vi "MBDRV_Communication With Server.vi"(8 "error in (no error)":errorcluster, 11 "Write To PLC":T4) -> (0 "error out":errorcluster, 3 "Read From PLC":T1)   [LabVIEW 2010]
uses:
  SubVIs/ModBUS Driver/Private/MBDRV_Command List.ctl
  SubVIs/ModBUS Driver/Private/MBDRV_Command Data.ctl
  SubVIs/ModBUS Driver/Private/MBDRV_Action.ctl
  SubVIs/ModBUS Driver/Private/MBDRV_Response List.ctl
  SubVIs/ModBUS Driver/Private/MBDRV_Response.ctl
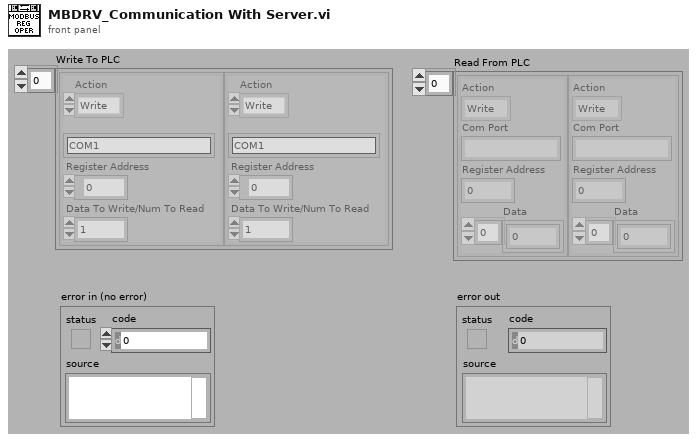
[diagram p1: front panel]
types:
  T1 = typedef "MBDRV_Response List.ctl" = T2[]
  T2 = typedef "MBDRV_Response.ctl" = cluster{"Action":T3, "Com Port":string, "Register Address":u16, "Data":i16[]}
  T3 = typedef "MBDRV_Action.ctl" = enum16{"Write", "Read"}
  T4 = typedef "MBDRV_Command List.ctl" = T5[]
  T5 = typedef "MBDRV_Command Data.ctl" = cluster{"Action":T3, "Com Port":string, "Register Address":u16, "Data To Write/Num To Read":i16}
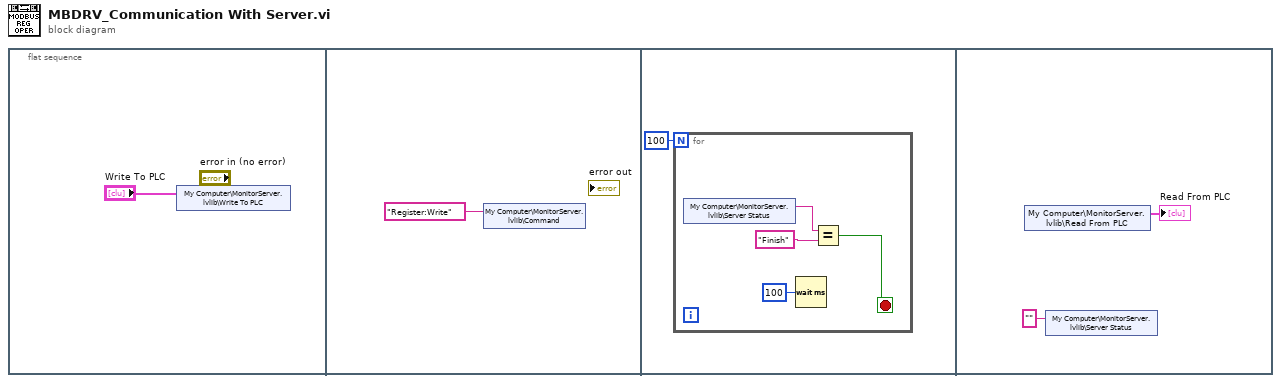
[diagram p0: block diagram]
diagram:
  n1 = flat-sequence {
    frame #0 {
      n2 = shared-variable "My Computer\\MonitorServer.lvlib\\Write To PLC"("Write To PLC") -> ()  [unwired: 1 in, 1 out]
    }
    frame #1 {
      n3 = shared-variable "My Computer\\MonitorServer.lvlib\\Command"("Register:Write" ("Command")) -> ()  [unwired: 1 in, 1 out]
    }
    frame #2 {
      n4 = for {
        N: 100 -> [_]
        stop <- w4 stop-if-true
        n5 = shared-variable "My Computer\\MonitorServer.lvlib\\Server Status"() -> (w7:string)  [unwired: 1 in, 1 out]
        n6 = Wait (ms)(milliseconds to wait=u32 100) -> ()  [unwired: 1 out]
        n7 = Equal?(x=w7, y="Finish") -> (x = y?=w4:bool)
      }
    }
    frame #3 {
      n8 = shared-variable "My Computer\\MonitorServer.lvlib\\Read From PLC"() -> (→"Read From PLC":T1)  [unwired: 1 in, 1 out]
      n9 = shared-variable "My Computer\\MonitorServer.lvlib\\Server Status"("" ("Server Status")) -> ()  [unwired: 1 in, 1 out]
    }
  }
